vi "StatTable_Prep.vi"(6 "Window Title":string, 7 "Path":path=path "C:/work/ADS1298/Modules/StatTable_Popup.vi", 8 "Table Row Hdrs[]":string[](array[string])=["ROW0", "ROW1", "ROW2"], 9 "Table Col Hdrs[]":string[](array[string])=["col1", "COL2", "COL3"], 11 "Table Data":string[][](array[string])) -> ()   [LabVIEW 2010]
uses:
  <vilib>/Utility/miscctls.llb/LVRectTypeDef.ctl
  <vilib>/Utility/miscctls.llb/LVPositionTypeDef.ctl
panel:
  in  "Bool Ctrl Offset":T1={"Left"=145, "Top"=40}
  in  "Table Ctrl Offset":T1={"Left"=25, "Top"=27}
  in  "Front Panel Base":T2={"Left"=0, "Top"=0, "Right"=140, "Bottom"=115}
  # "Constants (experimentally determined)"
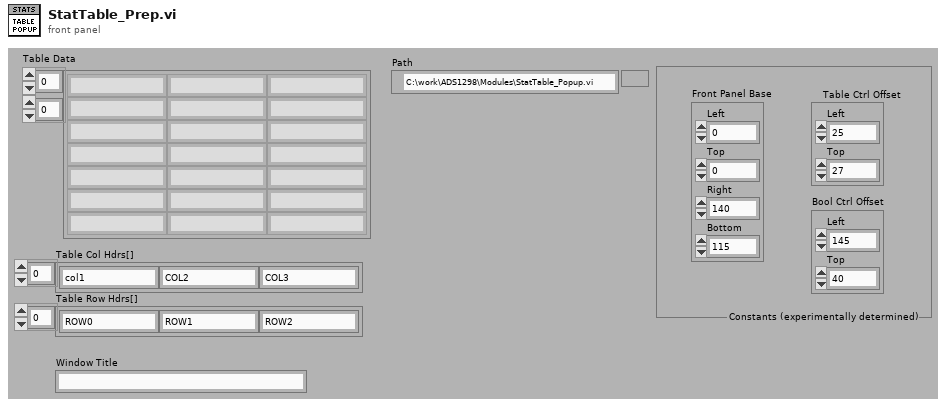
[diagram p1: front panel]
types:
  T1 = typedef "LVPositionTypeDef.ctl" = cluster{"Left":i32, "Top":i32}
  T2 = typedef "LVRectTypeDef.ctl" = cluster{"Left":i16, "Top":i16, "Right":i16, "Bottom":i16}
  T3 = enum16{"Open/Calc", "Setup Main Window", "Setup Table", "Setup Boolean", "Show VI"}
  T4 = enum32{"Invalid", "Standard", "Closed", "Hidden", "Minimized", "Maximized"}
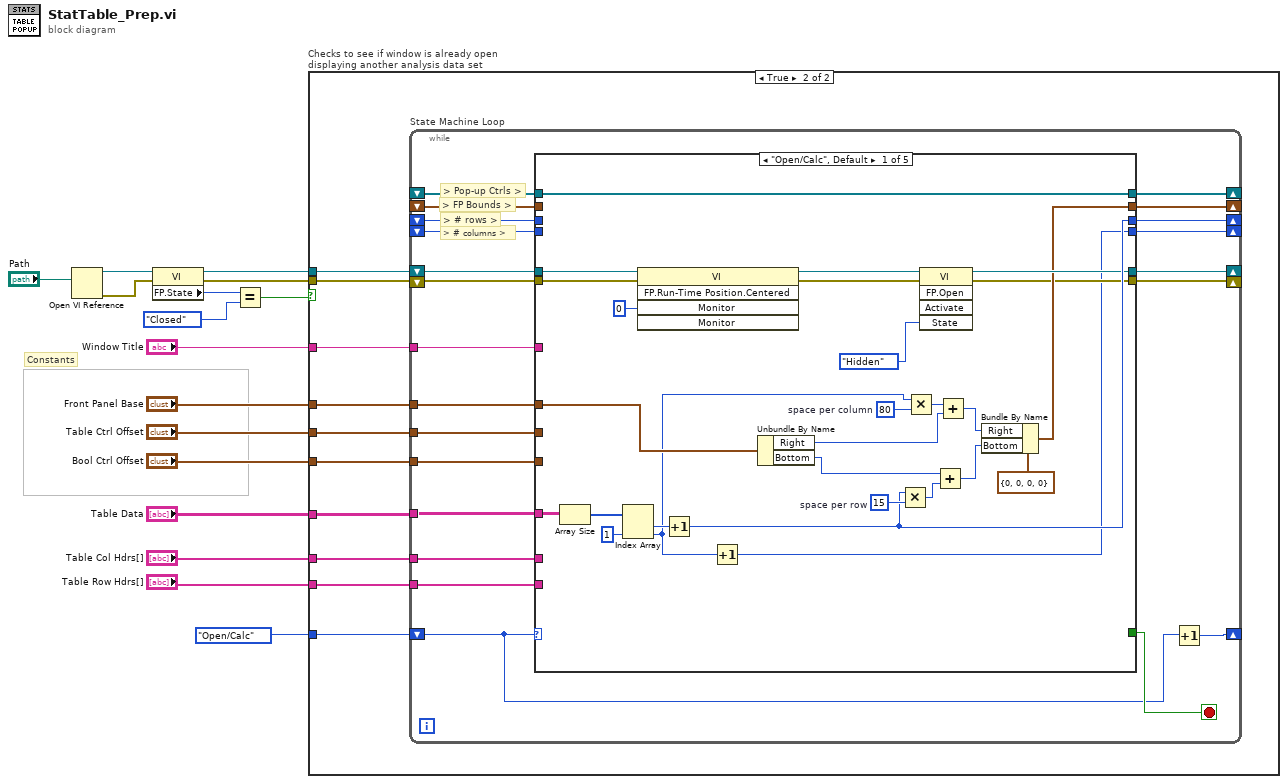
[diagram p0: block diagram]
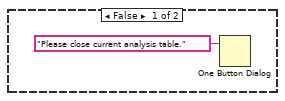
[diagram p2: hidden frame]
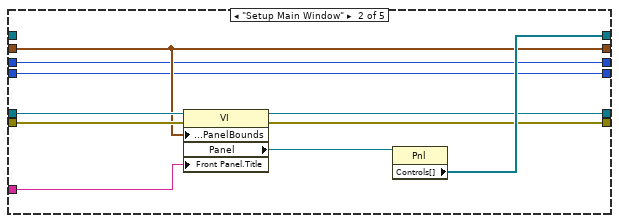
[diagram p3: hidden frame]
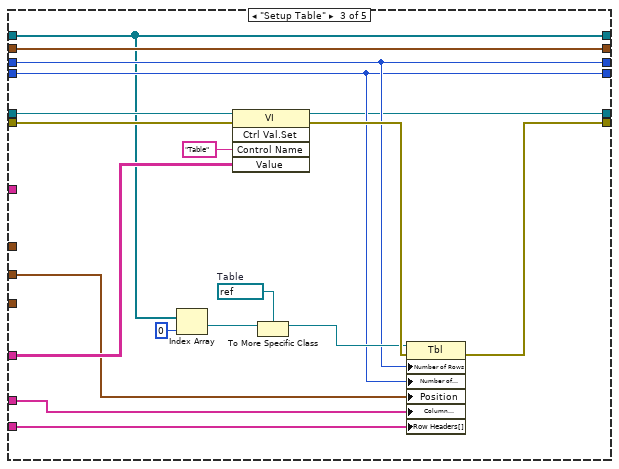
[diagram p4: hidden frame]
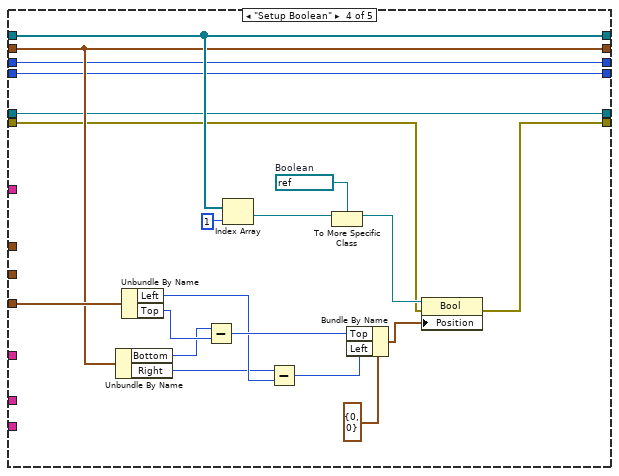
[diagram p5: hidden frame]
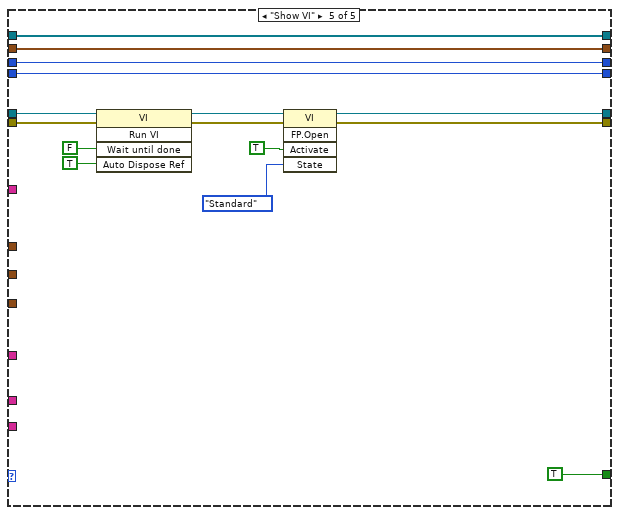
[diagram p6: hidden frame]
diagram:
  # "Constants"
  n1 = Open VI Reference(vi path="Path") -> (vi reference=w8:refnum<vi>, error out=w7:errorcluster)  [unwired: 2 in, 3 out]
  n2 = property class="VI"(reference=w8, error in=w7) -> (reference out=w6:refnum<vi>, error out=w5:errorcluster, "FP.State"=w4:T4)
  n3 = Equal?(x=w4, y=T4."Closed") -> (x = y?=w2:bool)
  n4 = case "Checks to see if window is already open displaying another analysis data set" shown="True" w2 {
    tunnel: "Table Data" -> [_ w27]
    tunnel: "Bool Ctrl Offset" -> [_ w26]
    tunnel: "Table Col Hdrs[]" -> [_ w25]
    tunnel: "Table Row Hdrs[]" -> [_ w24]
    tunnel: "Table Ctrl Offset" -> [_ w23]
    tunnel: "Front Panel Base" -> [_ w22]
    tunnel: w6 -> [_ w21]
    tunnel: "Window Title" -> [_ w20]
    tunnel: w5 -> [_ w19]
    tunnel: T3."Open/Calc" ("Enum") -> [_ w18]
    frame False {
      n5 = One Button Dialog(message="Please close current analysis table.") -> ()  [unwired: 2 out]
    }
    frame True {
      n6 = while "State Machine Loop" {
        tunnel: w27 -> [w49]
        tunnel: w26 -> [w36]
        tunnel: w25 -> [w35]
        tunnel: w24 -> [w34]
        tunnel: w23 -> [w37]
        tunnel: w22 -> [w48]
        shift-right: [w32] -> _
        shift-left: w21 -> [w47]
        shift-right: [w45] -> _
        shift-left: _ -> [w44]
        shift-right: [w43] -> _
        shift-left: _ -> [w42]
        shift-right: [w41] -> _
        shift-left: _ -> [w39]
        shift-right: [w40] -> _
        shift-left: _ -> [w38]
        shift-right: [w31] -> _
        shift-left: w18 -> [w30]
        tunnel: w20 -> [w29]
        shift-right: [w28] -> _
        shift-left: w19 -> [w46]
        stop <- w33 stop-if-true
        # "> Pop-up Ctrls >"
        # "> FP Bounds >"
        # "> # rows >"
        # "> # columns >"
        n7 = case shown="\"Open/Calc\", Default" w30 {
          tunnel: w49 -> [w76 _ w97 _ _]
          tunnel: w48 -> [w57 _ _ _ _]
          tunnel: w47 -> [w63 w82 w99 w109 w130]
          tunnel: w46 -> [w62 w81 w98 w105 w129]
          tunnel: [w58 w85 w89 w113 w131] -> w45
          tunnel: w44 -> [w58 _ w89 w113 w131]
          tunnel: [w55 w80 w90 w112 w132] -> w43
          tunnel: w42 -> [_ w80 w90 w112 w132]
          tunnel: [w60 w78 w92 w111 w133] -> w41
          tunnel: [w51 w79 w91 w110 w134] -> w40
          tunnel: w39 -> [_ w78 w92 w111 w133]
          tunnel: w38 -> [_ w79 w91 w110 w134]
          tunnel: w37 -> [_ _ w95 _ _]
          tunnel: w36 -> [_ _ _ w114 _]
          tunnel: w35 -> [_ _ w93 _ _]
          tunnel: w34 -> [_ _ w94 _ _]
          tunnel: [_ _ _ _ TRUE] -> w33
          tunnel: [w59 w84 w88 w109 w126] -> w32
          tunnel: w29 -> [_ w83 _ _ _]
          tunnel: [w52 w77 w87 w107 w125] -> w28
          frame "Open/Calc", Default {
            w64 = 15  # space per row
            w72 = 80  # space per column
            n8 = Array Size(array=w76) -> (size(s)=w75:i32[])
            n9 = Index Array(array=w75, index #2=1 ("index")) -> (element #1=w61:i32, element #2=w50:i32)  [unwired: 1 in]
            n10 = invoke class="VI" method="FP.Run-Time Position.Centered"(reference=w63, error in=w62, "Monitor"=i16 0) -> (reference out=w68:refnum<vi>, error out=w73:errorcluster)  [unwired: 2 in, 3 out]
            n11 = Increment(x=w61) -> (x+1=w60:i32)
            n12 = Increment(x=w50) -> (x+1=w51:i32)
            n13 = Unbundle By Name(w57) -> ("Right"=w70:i16, "Bottom"=w67:i16)
            n14 = Multiply(x=w60, y=w64) -> (x*y=w65:i32)
            n15 = Multiply(x=w50, y=w72) -> (x*y=w71:i32)
            n16 = invoke class="VI" method="FP.Open"(reference=w68, error in=w73, "State"=T4."Hidden") -> (reference out=w59:refnum<vi>, error out=w52:errorcluster)  [unwired: 2 in, 3 out]
            n17 = Add(x=w67, y=w65) -> (x+y=w66:i32)
            n18 = Add(x=w71, y=w70) -> (x+y=w69:i32)
            n19 = Bundle By Name(cluster=T2 {"Left"=0, "Top"=0, "Right"=0, "Bottom"=0} ("Front Panel Base"), "Right"=w69, "Bottom"=w66) -> (w55:T2)
          }
          frame "Setup Main Window" {
            n20 = property class="VI"(reference=w82, error in=w81, "Front Panel.PanelBounds"=w80, "Front Panel.Title"=w83) -> (reference out=w84:refnum<vi>, error out=w77:errorcluster, "Panel"=w86:refnum<vi>)
            n21 = property class="Pnl"(reference=w86) -> ("Controls[]"=w85:refnum<vi>[])  [unwired: 1 in, 2 out]
          }
          frame "Setup Table" {
            w103 = refnum<vi> refnum  # Table
            n22 = Index Array(array=w89, index=0) -> (element=w101:refnum<vi>)
            n23 = invoke class="VI" method="Ctrl Val.Set"(reference=w99, error in=w98, "Control Name"="Table", "Value"=w97) -> (reference out=w88:refnum<vi>, error out=w104:errorcluster)  [unwired: 1 in, 3 out]
            n24 = To More Specific Class(target class=w103, reference=w101) -> (specific class reference=w102:refnum<vi>)  [unwired: 1 in, 1 out]
            n25 = property class="Tbl"(reference=w102, error in=w104, "Number of Rows"=w92, "Number of Columns"=w91, "Position"=w95, "Column Headers[]"=w93, "Row Headers[]"=w94) -> (error out=w87:errorcluster)  [unwired: 1 out]
          }
          frame "Setup Boolean" {
            w121 = refnum<vi> refnum  # Boolean
            n26 = Unbundle By Name(w112) -> ("Bottom"=w123:i16, "Right"=w115:i16)
            n27 = Unbundle By Name(w114) -> ("Left"=w116:i32, "Top"=w124:i32)
            n28 = Subtract(x=w123, y=w124) -> (x-y=w117:i32)
            n29 = Index Array(array=w113, index=1) -> (element=w119:refnum<vi>)
            n30 = Subtract(x=w115, y=w116) -> (x-y=w118:i32)
            n31 = To More Specific Class(target class=w121, reference=w119) -> (specific class reference=w106:refnum<vi>)  [unwired: 1 in, 1 out]
            n32 = Bundle By Name(cluster=T1 {"Left"=0, "Top"=0} ("Bool Ctrl Offset"), "Top"=w117, "Left"=w118) -> (w122:T1)
            n33 = property class="Bool"(reference=w106, error in=w105, "Position"=w122) -> (error out=w107:errorcluster)  [unwired: 1 out]
          }
          frame "Show VI" {
            n34 = invoke class="VI" method="Run VI"(reference=w130, error in=w129, "Wait until done"=FALSE ("Wait Until Done"), "Auto Dispose Ref"=TRUE ("Auto Dispose Reference")) -> (reference out=w128:refnum<vi>, error out=w127:errorcluster)  [unwired: 1 in, 3 out]
            n35 = invoke class="VI" method="FP.Open"(reference=w128, error in=w127, "Activate"=TRUE ("Activate?"), "State"=T4."Standard") -> (reference out=w126:refnum<vi>, error out=w125:errorcluster)  [unwired: 1 in, 3 out]
          }
        }
        n36 = Increment(x=w30) -> (x+1=w31:T3)
      }
    }
  }
